vi "Set Interface.vi"(8 "error in (no error)":errorcluster, 10 "interface":tag, 11 "Thread Configuration in":refnum<class "Thread Configuration.lvclass">) -> (0 "error out":errorcluster, 3 "Thread Configuration out":refnum<class "Thread Configuration.lvclass">)   [LabVIEW 2017, in "PXImc.lvlib" / "Thread Configuration.lvclass"]
uses:
  Thread Configuration.lvclass
  Thread Configuration.lvclass/Thread Configuration.ctl
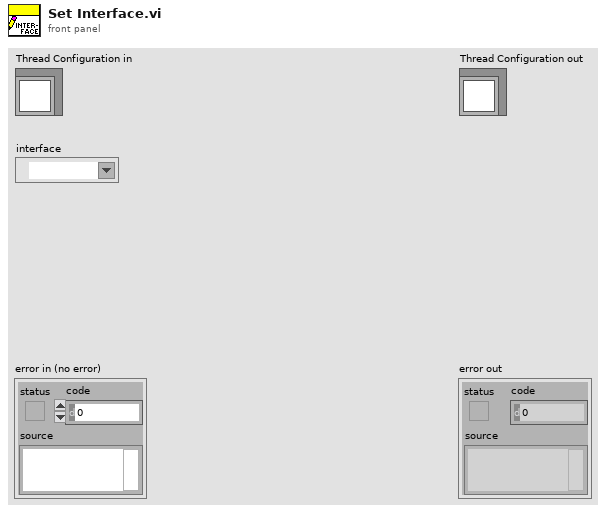
[diagram p1: front panel]
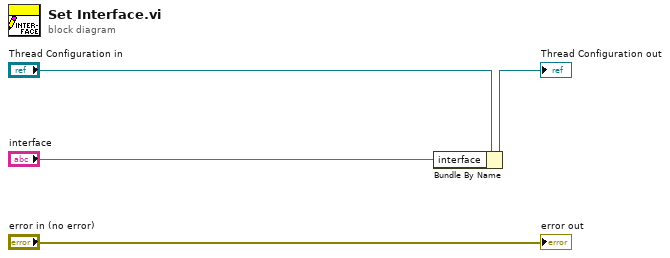
[diagram p0: block diagram]
diagram:
  n1 = Bundle By Name(cluster="Thread Configuration in", "interface"="interface") -> (→"Thread Configuration out":refnum<class "Thread Configuration.lvclass">)
  "error out" <- "error in (no error)"
